vi "GetPathToAppPlugin.vi"(8 "ErrorArray In":errorcluster[](array[cluster]), 11 "Bus.lvclass In":refnum<class "Bus.lvclass">) -> (0 "ErrorArray Out":errorcluster[](array[cluster]), 2 "AppPluginINIFilePath":path, 3 "Bus.lvclass Out":refnum<class "Bus.lvclass">)   [LabVIEW 2014]
uses:
  Bus.lvclass
  Bus.lvclass/Bus.ctl
  Accessors/Read AppModuleID.vi
  <vilib>/Utility/error.llb/Error Cluster From Error Code.vi
  <vilib>/ErrorRing/Error Ring.xnode
  <userlib>/NIST/NISTErrorLib/NISTErrorLib.lvlib
  Applications/AppModule/AppModule.lvlib
  Applications/AppPlugins/AppPluginBaseClass/AppPluginsBase.lvclass
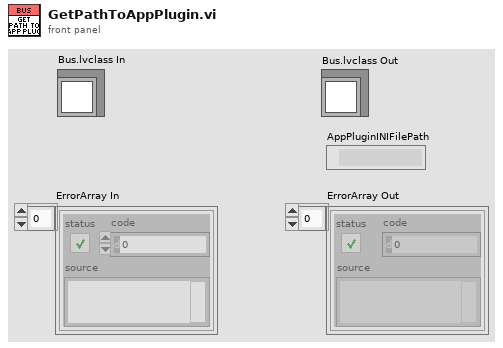
[diagram p1: front panel]
types:
  T1 = typedef "AppModule.lvlib/clBroadcastEvents.ctl" = cluster{"DidInit":refnum<user-event>, "StatusUpdate":refnum<user-event>, "ErrorReport":refnum<user-event>, "DidStop":refnum<user-event>, "PathToINI":refnum<user-event>, "InputData":refnum<user-event>, "OutputData":refnum<user-event>, "BcAppInfo":refnum<user-event>, "ConfigData":refnum<user-event>}
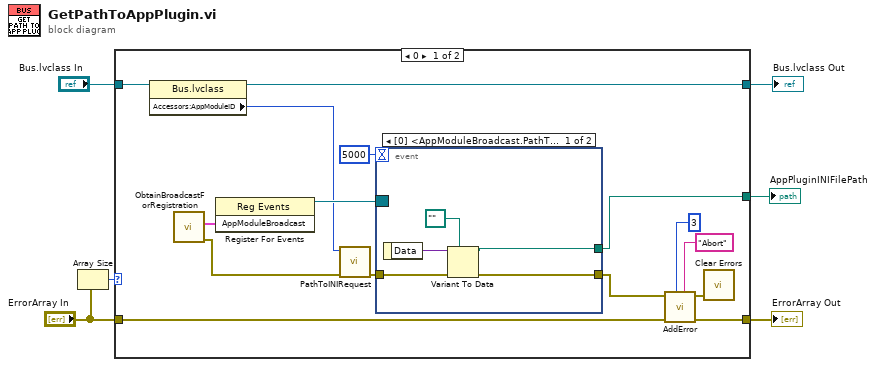
[diagram p0: block diagram]
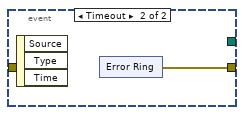
[diagram p2: hidden frame]
diagram:
  n1 = Array Size(array="ErrorArray In") -> (size(s)=w5:i32)
  n2 = case shown="0" w5 {
    tunnel: "ErrorArray In" -> [w21 w34]
    tunnel: [w20 w34] -> w6
    tunnel: "Bus.lvclass In" -> [w16 w33]
    tunnel: [w10 w33] -> w2
    tunnel: [w9 _] -> w1
    frame 0 {
      n3 = property class="Bus.lvclass"(reference=w16) -> (reference out=w10:refnum<class "Bus.lvclass">, "Accessors:AppModuleID"=w11:i32)  [unwired: 1 in, 1 out]
      n4 = call "ObtainBroadcastForRegistration.vi"() -> ("error out"=w13:errorcluster, "AppModuleBroadcast"=w15:T1)  [unwired: 10 in]
      n5 = register-events(w15) -> (reference out=w14:refnum<event-registration>)  [unwired: 2 in, 1 out]
      n6 = call "PathToINIRequest.vi"("error in (no error)"=w13, "ModuleID"=w11) -> ("error out"=w12:errorcluster)  [unwired: 9 in]
      n7 = event shown="[0] <AppModuleBroadcast.PathToINI>: User Event" {
        selector: w14 -> [_ _]
        dyn-events: _ -> [_ _]
        timeout: 5000 -> [_ _]
        tunnel: w12 -> [w25 _]
        tunnel: [w22 _] -> w9
        tunnel: [w24 w27] -> w8
        event User Event {
          n8 = event-data() -> ("Data"=w26:variant)  [unwired: 1 in]
          n9 = Variant To Data(error in=w25, type=path "", Variant=w26) -> (data=w22:path, error out=w24:errorcluster)
        }
        event Timeout {
          n10 = event-data() -> ()  [unwired: 1 in, 3 out]
          n11 = xnode "Error Ring"() -> ("error out"=w27:errorcluster)
        }
      }
      n12 = call <userlib>:"AddError.vi"("Severity"="Abort" ("String"), "Priority"=u8 3, "ErrorArray"=w21, "error in (no error)"=w8) -> ("ErrorArray"=w20:errorcluster[], "error out"=w19:errorcluster)  [unwired: 6 in]
      n13 = call <vilib>:"Clear Errors.vi"("error in (no error)"=w19) -> ()  [unwired: 5 in, 2 out]
    }
    frame 1, Default {
    }
  }
  "ErrorArray Out" <- w6
  "Bus.lvclass Out" <- w2
  "AppPluginINIFilePath" <- w1
